vi "Init_All_AE.vi"(7 "Flat File Path":path=path "C:/Users/STED/Desktop/Cambridge STED Control Software/Host VIs/SLM/Flatness Correction LSH0700935/CAL_LSH0700935_770nm.bmp", 8 "HoloArray In":T1[](array[typedef]) {"Modes"."Amplititute" step=0.05}, 11 "General settings":T2={"Holo size (pixels)"=300, "Top hat radius"=0.5, "Number of modes"=20, "Bkg gradient X"=-40.0, "Bkg gradient Y"=-40.0, "Flat"=FALSE, "Mode Matrix"=0}) -> (0 "Holo Array Out":T1[](array[typedef]) {"Modes"."Amplititute" step=0.05})   [LabVIEW 2014]
uses:
  Controls/Holo Controls.ctl
  Controls/SLM General Settings.ctl
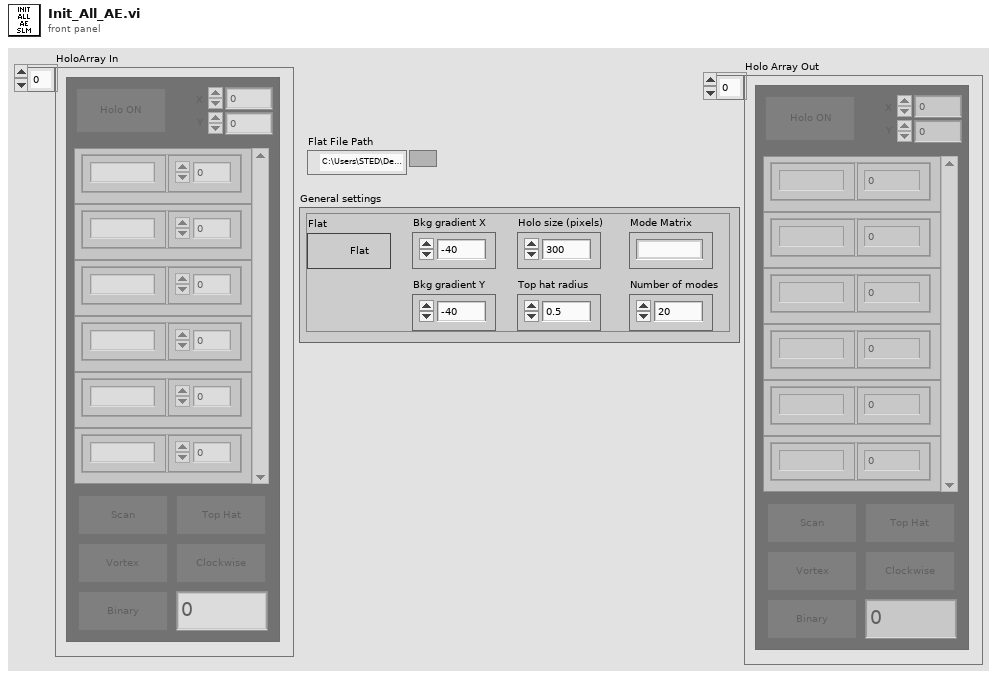
[diagram p1: front panel]
types:
  T1 = typedef "Holo Controls.ctl" = cluster{"Top Hat":bool, "Modes":cluster{"Mode ID":string, "Amplititute":dbl}[], "Vortex":bool, "Clockwise":bool, "X":dbl, "Y":dbl, "Holo ON":bool, "Scan":bool, "Binary":bool, "Binary Angle":dbl}
  T2 = typedef "SLM General Settings.ctl" = cluster{"Holo size (pixels)":i32, "Top hat radius":dbl, "Number of modes":i32, "Bkg gradient X":dbl, "Bkg gradient Y":dbl, "Flat":bool, "Mode Matrix":u16}
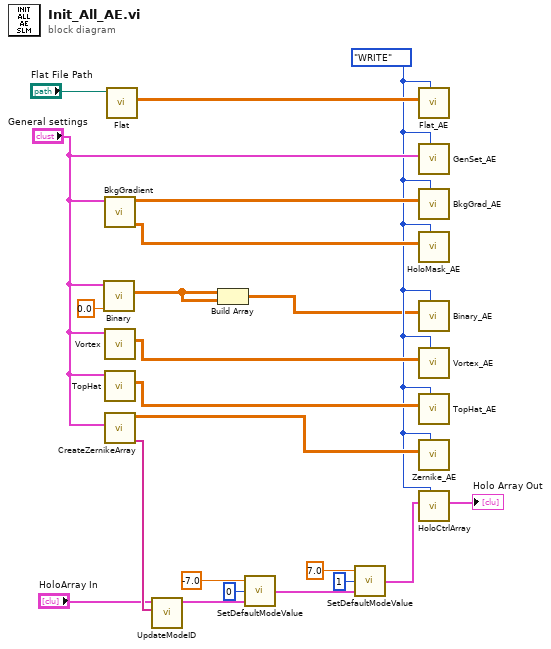
[diagram p0: block diagram]
diagram:
  w3 = enum16{"READ", "WRITE"}."WRITE" ("Action")
  n1 = call "Binary.vi"("Angle"=0.0, "General settings"="General settings") -> ("Binary"=w2:dbl[][])  [unwired: 9 in]
  n2 = call "BkgGradient.vi"("General settings"="General settings") -> ("Holo mask"=w15:dbl[][], "gradient"=w14:dbl[][])  [unwired: 9 in]
  n3 = call "Vortex.vi"("General settings"="General settings") -> ("Vortex"=w19:dbl[][])  [unwired: 10 in]
  n4 = call "TopHat.vi"("General settings"="General settings") -> ("TopHat"=w18:dbl[][])  [unwired: 10 in]
  n5 = call "CreateZernikeArray.vi"("General settings"="General settings") -> ("Mode IDs"=w16:string[], "Modes Out"=w17:dbl[][][])  [unwired: 9 in]
  n6 = call "Flat.vi"("File Path"="Flat File Path") -> ("Flatness"=w22:dbl[][])  [unwired: 10 in]
  n7 = call "UpdateModeID.vi"("Mode IDs"=w16, "Array in"="HoloArray In") -> ("Array out"=w13:T1[])  [unwired: 9 in]
  n8 = Build Array(w2, w2) -> (w1:dbl[][][])
  n9 = call "SetDefaultModeValue.vi"("Array in"=w13, "index"=0, "Amplititute"=-7.0) -> ("output array"=w10:T1[])
  n10 = call "SetDefaultModeValue.vi"("Array in"=w10, "index"=1, "Amplititute"=7.0) -> ("output array"=w7:T1[])
  n11 = call "Flat_AE.vi"("Action"=w3, "Flat In"=w22) -> ()  [unwired: 9 in, 1 out]
  n12 = call "GenSet_AE.vi"("Enum"=w3, "General settings"="General settings") -> ()  [unwired: 9 in, 1 out]
  n13 = call "BkgGrad_AE.vi"("Action"=w3, "BkgGrad In"=w14) -> ()  [unwired: 9 in, 1 out]
  n14 = call "HoloMask_AE.vi"("Action"=w3, "HoloMask In"=w15) -> ()  [unwired: 9 in, 1 out]
  n15 = call "Binary_AE.vi"("Action"=w3, "BINARY In"=w1) -> ()  [unwired: 9 in, 1 out]
  n16 = call "Vortex_AE.vi"("Action"=w3, "Vortex In"=w19) -> ()  [unwired: 9 in, 1 out]
  n17 = call "TopHat_AE.vi"("Action"=w3, "TopHat In"=w18) -> ()  [unwired: 9 in, 1 out]
  n18 = call "Zernike_AE.vi"("Action"=w3, "Zernike In"=w17) -> ()  [unwired: 9 in, 1 out]
  n19 = call "HoloCtrlArray.vi"("Action"=w3, "Holo Array In"=w7) -> ("Holo Array Out"=→"Holo Array Out":T1[])  [unwired: 9 in]
